vi "Populate Mag Lab Hardware List.vi"(4 "Seconds between samples":dbl=1.0 format="%_4f", 6 "Channels to scan (empty - don't use scanner option)":i32[](array[numeric]), 8 "error in (no error)":errorcluster, 11 "VISA Resourse Names":refnum<visa-resource-name>[](array[refnum])) -> (0 "error out":errorcluster, 2 "Names":string[](array[string]), 3 "Instrument List":refnum<class "Mag Lab Hardware.lvclass">[](array[class]))   [LabVIEW 2015]
uses:
  Mag Lab Hardware.lvclass
  OO Devices/Device/Device type.ctl
  Cryo-Con/Cryo-Con.lvclass
  HP/HP87NN/HP87NN.lvclass
  HP/HPNetworkAnalyzer/HPNeworkAnalyzer.lvclass
  Linear Research/Linear Research.lvclass
  HP Counter/HP counter.lvclass
  LakeShore/Lake Shore Temperature Controller/LakeShore T Controller.lvclass
  LakeShore/LakeShore370/LakeShore370.lvclass
  Keithley/Keithley Meter/Keithley Meter.lvclass
  Keithley/Keithley Meter/Keithley Meter.lvclass/Keithley Meter.ctl
  Oxford/Power supply/Oxford Power Supply.lvclass
  Oxford/Mercury IPS/Oxford Mercury IPS.lvclass
  Neocera/Neocera.lvclass
  Keithley/Keithley Current Source/Keithley Current Source.lvclass
  Stanford Research/Stanford Research.lvclass
  Keithley/Keithley 182/Keithley 182 Folder/Keithley 182.lvclass
  Mag Lab Root/Mag Lab Root.lvclass/Mag Lab Root.ctl
  Mag Lab Hardware.lvclass/Mag Lab Hardware.ctl
  Keithley/Keithley Meter/Write Source-meter.vi
  Mag Lab Root/Mag Lab Root.lvclass
panel:
  in  "Instrument":T1=enum."LkShr 340 chA&B"
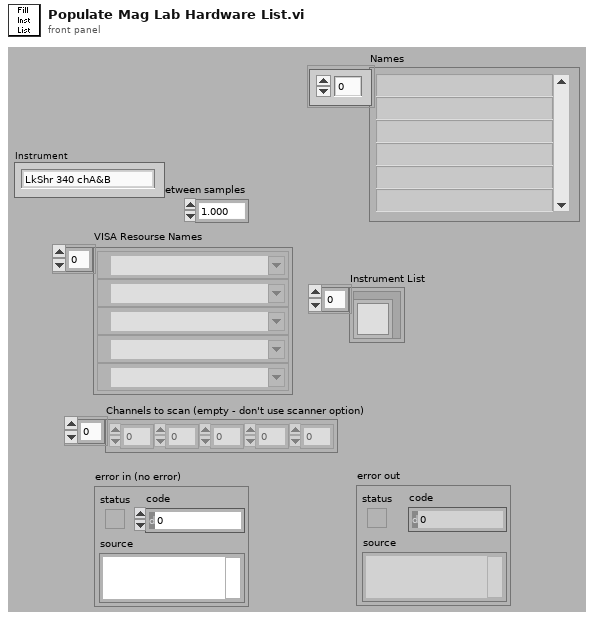
[diagram p1: front panel]
types:
  T1 = typedef "Device type.ctl" = enum16{"NONE", "Neocera 21", "LakeShore 335", "LakeShore 340", "LkShr 340 chA&B", "LakeShore 370", "SRS 850", "SRS 830", "LR 700", "EG&G 5302", "EG&G 7260", "EG&G 7280", "AH 2500", "Keithley meter", "Keithley electrometer", "Keithley 182", "HP 5385", "HP 53181", "HP 53132", "ITC503", "IPS120", "Oxford Mercury IPS", "Oxford PS", "Test", "DC Facility Magnet", "Cryomagnetics PS", "Keithley 2400", "Keithley current source", "Cryo-Con 22C", "HP87NN", "HP4395A"}
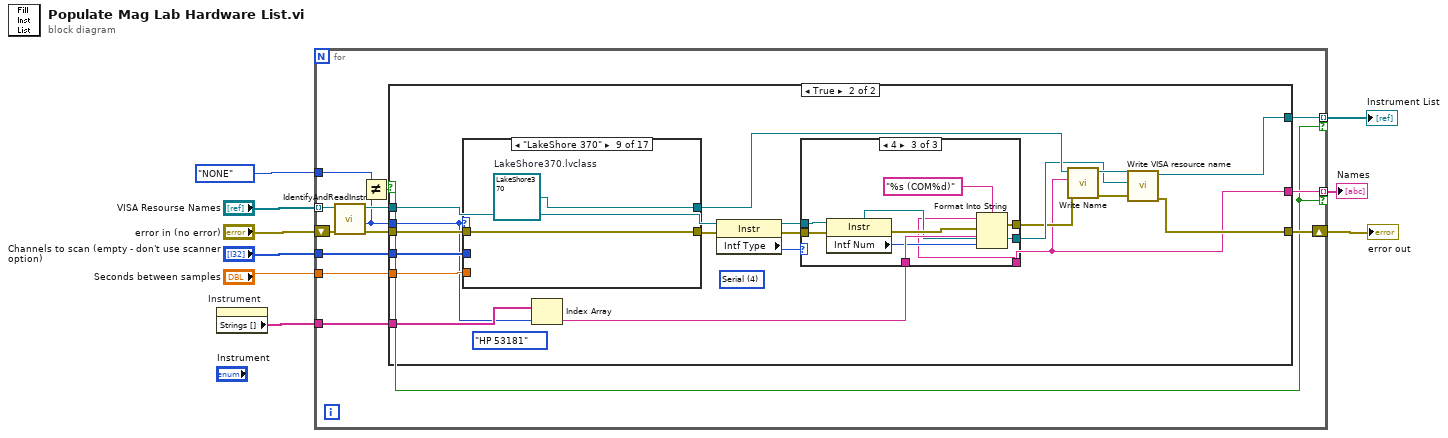
[diagram p0: block diagram]
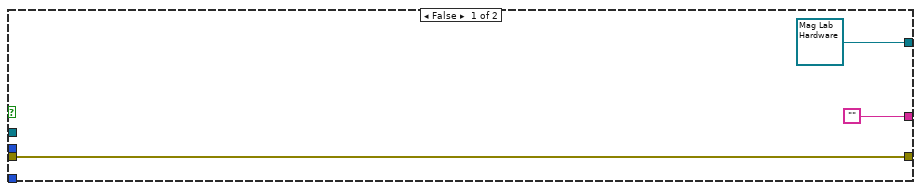
[diagram p2: hidden frame]
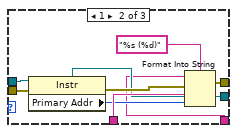
[diagram p4: hidden frame]
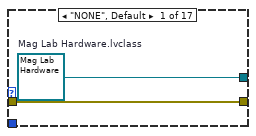
[diagram p5: hidden frame]
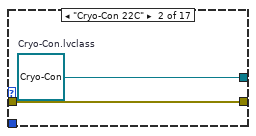
[diagram p6: hidden frame]
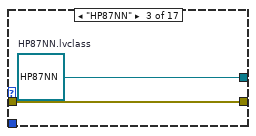
[diagram p7: hidden frame]
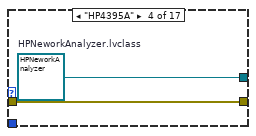
[diagram p8: hidden frame]
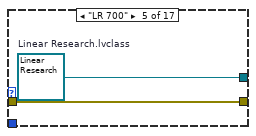
[diagram p9: hidden frame]
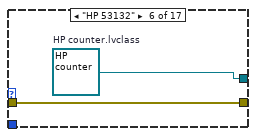
[diagram p10: hidden frame]
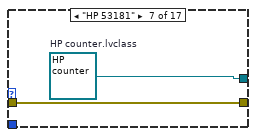
[diagram p11: hidden frame]
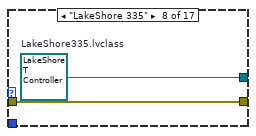
[diagram p12: hidden frame]
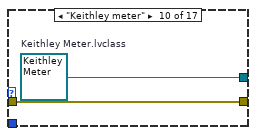
[diagram p13: hidden frame]
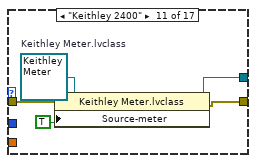
[diagram p14: hidden frame]
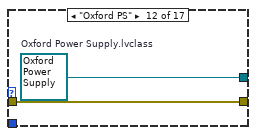
[diagram p15: hidden frame]
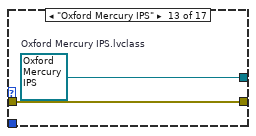
[diagram p16: hidden frame]
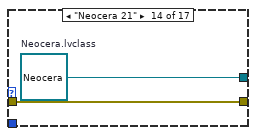
[diagram p17: hidden frame]
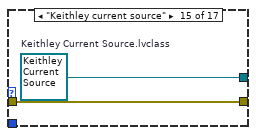
[diagram p18: hidden frame]
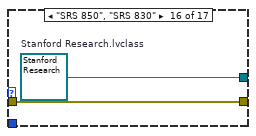
[diagram p19: hidden frame]
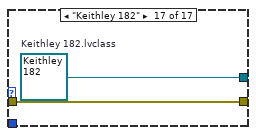
[diagram p20: hidden frame]
diagram:
  n1 = property on="Instrument" class="Enum (strict)"() -> ("Strings []"=w4:string[])  [unwired: 2 in, 2 out]
  n2 = for {
    tunnel: "VISA Resourse Names" -> [w20] mode=indexing
    shift-right: [w16] -> w7
    shift-left: "error in (no error)" -> [w22]
    tunnel: "Channels to scan (empty - don't use scanner option)" -> [w19]
    tunnel: "Seconds between samples" -> [w18]
    tunnel: w4 -> [w13]
    tunnel: Device_type."NONE" ("Instrument") -> [w15]
    tunnel: [w12] -> w2 mode=indexing if=w10
    tunnel: [w11] -> w1 mode=indexing if=w10
    n3 = call "IdentifyAndReadInstr.vi"("error in (no error)"=w22, "VISA Resource Name"=w20) -> ("error out"=w21:errorcluster, "Instrument"=w14:T1, "VISA Resource Name Out"=w17:refnum<visa-resource-name>)  [unwired: 7 out]
    n4 = Not Equal?(x=w15, y=w14) -> (x != y?=w10:bool)
    n5 = case shown="True" w10 {
      tunnel: w21 -> [w25 w44]
      tunnel: w19 -> [_ w43]
      tunnel: w18 -> [_ w42]
      tunnel: w17 -> [_ w37]
      tunnel: w14 -> [_ w39]
      tunnel: [refnum<class "Mag Lab Hardware.lvclass"> refnum ("Mag Lab Hardware out") w27] -> w12
      tunnel: [w25 w28] -> w16
      tunnel: w13 -> [_ w41]
      tunnel: ["" w26] -> w11
      frame False {
      }
      frame True {
        (unwired) Device_type."HP 53181" ("Instrument")
        (unwired) u16 4 items=["GPIB"=1, "VXI"=2, "GPIB-VXI"=3, "Serial"=4, "PXI"=5, "TCPIP"=6, "USB"=7, "FireWire"=9] ("Interface Information:Interface Type")
        n6 = case shown="\"LakeShore 370\"" w39 {
          tunnel: w44 -> [w67 w69 w71 w73 w75 w77 w79 w81 w83 w85 w88 w92 w94 w96 w98 w100 w102]
          tunnel: [w67 w69 w71 w73 w75 w77 w79 w81 w83 w85 w86 w92 w94 w96 w98 w100 w102] -> w36
          tunnel: [w66 w68 w70 w72 w74 w76 w78 w80 w82 w84 w89 w91 w93 w95 w97 w99 w101] -> w33
          tunnel: w43 -> [_ _ _ _ _ _ _ _ _ _ _ _ _ _ _ _ _]
          tunnel: w42 -> [_ _ _ _ _ _ _ _ _ _ _ _ _ _ _ _ _]
          frame "NONE", Default {
            w66 = refnum<class "Mag Lab Hardware.lvclass"> refnum  # Mag Lab Hardware.lvclass
          }
          frame "Cryo-Con 22C" {
            w68 = refnum<class "Cryo-Con.lvclass"> refnum  # Cryo-Con.lvclass
          }
          frame "HP87NN" {
            w70 = refnum<class "HP87NN.lvclass"> refnum  # HP87NN.lvclass
          }
          frame "HP4395A" {
            w72 = refnum<class "HPNeworkAnalyzer.lvclass"> refnum  # HPNeworkAnalyzer.lvclass
          }
          frame "LR 700" {
            w74 = refnum<class "Linear Research.lvclass"> refnum  # Linear Research.lvclass
          }
          frame "HP 53132" {
            w76 = refnum<class "HP counter.lvclass"> refnum  # HP counter.lvclass
          }
          frame "HP 53181" {
            w78 = refnum<class "HP counter.lvclass"> refnum  # HP counter.lvclass
          }
          frame "LakeShore 335" {
            w80 = refnum<class "LakeShore T Controller.lvclass"> refnum  # LakeShore335.lvclass
          }
          frame "LakeShore 370" {
            w82 = refnum<class "LakeShore370.lvclass"> refnum  # LakeShore370.lvclass
          }
          frame "Keithley meter" {
            w84 = refnum<class "Keithley Meter.lvclass"> refnum  # Keithley Meter.lvclass
          }
          frame "Keithley 2400" {
            w90 = refnum<class "Keithley Meter.lvclass"> refnum  # Keithley Meter.lvclass
            n7 = property class="Keithley Meter.lvclass"(reference=w90, error in=w88, "Source-meter"=TRUE) -> (reference out=w89:refnum<class "Keithley Meter.lvclass">, error out=w86:errorcluster)
          }
          frame "Oxford PS" {
            w91 = refnum<class "Oxford Power Supply.lvclass"> refnum  # Oxford Power Supply.lvclass
          }
          frame "Oxford Mercury IPS" {
            w93 = refnum<class "Oxford Mercury IPS.lvclass"> refnum  # Oxford Mercury IPS.lvclass
          }
          frame "Neocera 21" {
            w95 = refnum<class "Neocera.lvclass"> refnum  # Neocera.lvclass
          }
          frame "Keithley current source" {
            w97 = refnum<class "Keithley Current Source.lvclass"> refnum  # Keithley Current Source.lvclass
          }
          frame "SRS 850", "SRS 830" {
            w99 = refnum<class "Stanford Research.lvclass"> refnum  # Stanford Research.lvclass
          }
          frame "Keithley 182" {
            w101 = refnum<class "Keithley 182.lvclass"> refnum  # Keithley 182.lvclass
          }
        }
        n8 = Index Array(array=w41, index=w39) -> (element=w40:string)
        n9 = property class="Instr"(reference=w37, error in=w36) -> (reference out=w38:refnum<visa-resource-name>, error out=w35:errorcluster, "Intf Type"=w34:u16)
        n10 = case shown="4" w34 {
          tunnel: w40 -> [w45 w54 w63]
          tunnel: [w46 w52 w61] -> w31
          tunnel: [w45 w51 w60] -> w26
          tunnel: [w47 w50 w59] -> w30
          tunnel: w38 -> [w46 w49 w58]
          tunnel: w35 -> [w47 w48 w57]
          frame 0, Default {
          }
          frame 1 {
            n11 = property class="Instr"(reference=w49, error in=w48) -> (reference out=w52:refnum<visa-resource-name>, error out=w56:errorcluster, "Primary Addr"=w53:u16)
            n12 = Format Into String(format string="%s (%d)", error in=w56, w54, w53) -> (resulting string=w51:string, error out=w50:errorcluster)  [unwired: 1 in]
          }
          frame 4 {
            n13 = property class="Instr"(reference=w58, error in=w57) -> (reference out=w61:refnum<visa-resource-name>, error out=w65:errorcluster, "Intf Num"=w62:u16)
            n14 = Format Into String(format string="%s (COM%d)", error in=w65, w63, w62) -> (resulting string=w60:string, error out=w59:errorcluster)  [unwired: 1 in]
          }
        }
        n15 = call "Write Name.vi"("error in (no error)"=w30, "Name"=w26, "Mag Lab Root in"=w33) -> ("error out"=w29:errorcluster, "Mag Lab Root out"=w32:refnum<class "Mag Lab Hardware.lvclass">)  [unwired: 7 in]
        n16 = call "Write VISA resource name.vi"("error in (no error)"=w29, "VISA resource name"=w31, "Mag Lab Hardware in"=w32) -> ("error out"=w28:errorcluster, "Mag Lab Hardware out"=w27:refnum<class "Mag Lab Hardware.lvclass">)  [unwired: 7 in]
      }
    }
  }
  "error out" <- w7
  "Instrument List" <- w2
  "Names" <- w1
